vi "Get Unit Quaternion.vi"(1 "quaternion":T1) -> (0 "unit quaternion":T1)   [LabVIEW 2017, in "NI_Kinematics.lvlib"]
doc: "Computes the unit quaternion of a quaternion.\n\n<B>.m file:</B> unit"
uses:
  <vilib>/robotics/Kinematics/NI_Kinematics.lvlib
  <vilib>/robotics/Kinematics/Quaternion.ctl
  <vilib>/Analysis/_algsub.llb/Real Vector Norm.vi
  <vilib>/Analysis/NI_AALPro.lvlib
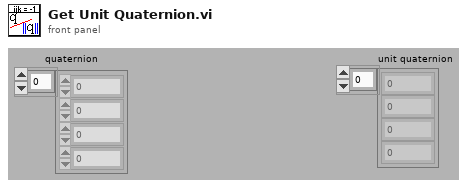
[diagram p1: front panel]
types:
  T1 = typedef "NI_Kinematics.lvlib/Quaternion.ctl" = dbl[]
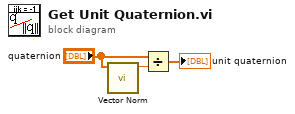
[diagram p0: block diagram]
diagram:
  n1 = call-poly <vilib>:"Vector Norm.vi"("Input Vector"="quaternion") -> ("norm"=w3:dbl)  [unwired: 2 in, 8 out]
  n2 = Divide(x="quaternion", y=w3) -> (x/y=→"unit quaternion":T1)
